vi "LogicGates.vi"() -> ()   [LabVIEW 2020]
panel:
  out "not 4":bool
  in  "Boolean 3":bool
  out "XOR":bool
  in  "Boolean 2":bool
  in  "Boolean":bool
  out "OR":bool
  in  "OR 2":bool
  in  "OR1":bool
  out "AND":bool
  in  "AND 2":bool
  in  "AND1":bool
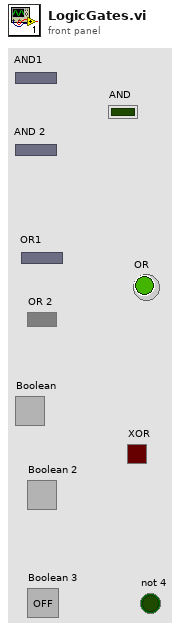
[diagram p1: front panel]
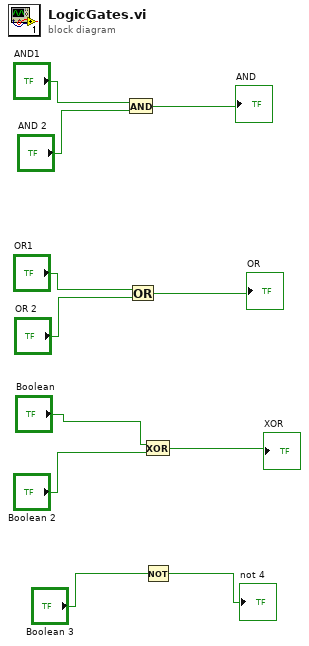
[diagram p0: block diagram]
diagram:
  n1 = And(x="AND1", y="AND 2") -> (x .and. y?=→"AND":bool)
  n2 = Or(x="OR1", y="OR 2") -> (x .or. y?=→"OR":bool)
  n3 = Exclusive Or(1:"Boolean 2", 2:"Boolean") -> (0:→"XOR":bool)
  n4 = Not(x="Boolean 3") -> (.not. x?=→"not 4":bool)
